vi "TransducerStartCalibration.vi"(8 "error in (no error)":errorcluster, 11 "Connection Data In":T1) -> (0 "error out":errorcluster, 3 "Connection Data Out":T1)   [LabVIEW 2014, in "MSX-E3701_dll.lvlib"]
uses:
  MSX-E3701_dll.lvlib
  E:/Repositorio Magnis/INF002/v0/Modules/HAL/Drivers/Sync/ADDI-DATA MSX-E3701/API/MX370x.dll
  MX370x.dll
  Typedef/Connection Data.ctl
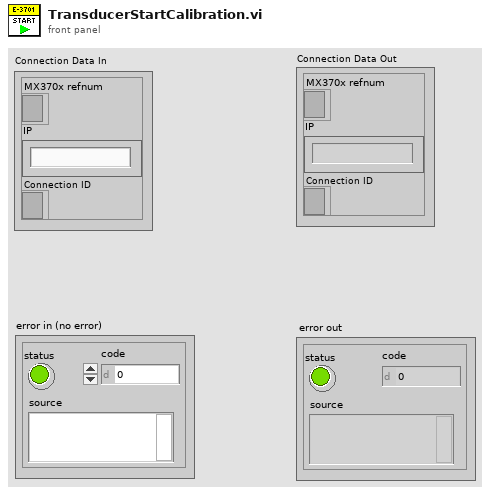
[diagram p1: front panel]
types:
  T1 = typedef "MSX-E3701_dll.lvlib/Connection Data.ctl" = cluster{"MX370x refnum":refnum<k24>, "IP":string, "Connection ID ":refnum<k5>}
  T2 = typedef "MSX-E3701_dll.lvlib/Calibration Data.ctl" = cluster{"Type":u64, "Impedance":u64, "Frequency":u64, "Veff":dbl, "Sensibility":dbl, "Range":dbl, "Transducer selection index":u64, "Name":string, "Calibration status":u64, "Calibration Channel":u64, "Stop Button":bool}
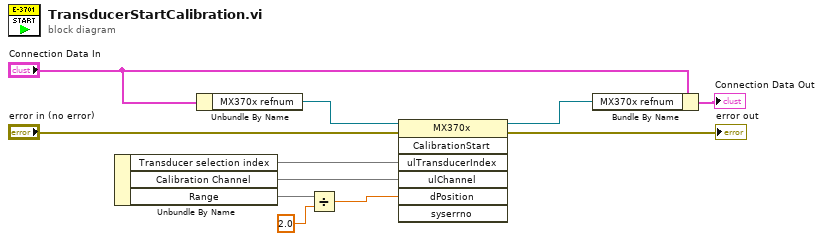
[diagram p0: block diagram]
diagram:
  n1 = Unbundle By Name() -> (w6:T2, "Transducer selection index"=w2, "Calibration Channel"=w1, "Range"=w5)
  n2 = Unbundle By Name("Connection Data In") -> ("MX370x refnum"=w12:refnum<k24>)
  n3 = Divide(x=w5, y=2.0) -> (x/y=w4:dbl)
  n4 = invoke class="MX370x" method="CalibrationStart"(reference=w12, error in="error in (no error)", "ulTransducerIndex"=w2, "ulChannel"=w1, "dPosition"=w4) -> (reference out=w8:refnum<k24>, error out=→"error out":errorcluster)  [unwired: 2 in, 5 out]
  n5 = Bundle By Name(cluster="Connection Data In", "MX370x refnum"=w8) -> (→"Connection Data Out":T1)
